vi "TemperatureSensor.vi"() -> (3 "Output":u64)   [LabVIEW 2014]
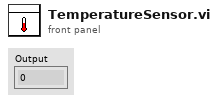
[diagram p1: front panel]
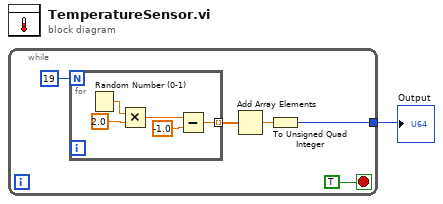
[diagram p0: block diagram]
diagram:
  n1 = while {
    tunnel: [w3] -> w1
    stop <- TRUE stop-if-true
    n2 = for {
      N: 19 -> [_]
      tunnel: [w7] -> w6 mode=indexing
      n3 = Random Number (0-1)() -> (number: 0 to 1=w10:dbl)
      n4 = Multiply(x=w10, y=2.0) -> (x*y=w8:dbl)
      n5 = Subtract(x=w8, y=-1.0) -> (x-y=w7:dbl)
    }
    n6 = Add Array Elements(numeric array=w6) -> (sum=w4:dbl)
    n7 = To Unsigned Quad Integer(1:w4) -> (0:w3:u64)
  }
  "Output" <- w1
